vi "teste 9142.vi"() -> ()   [LabVIEW 2018]
uses:
  <vilib>/Instr/_visa.llb/VISA Configure Serial Port (Serial Instr).vi
panel:
  in  "OK Button":bool
  out "read buffer":string
  in  "stop":bool
  in  "Boolean":bool
  in  "read buffer 2":string
  out "error out 2":errorcluster
  in  "VISA resource name":refnum<visa-resource-name>
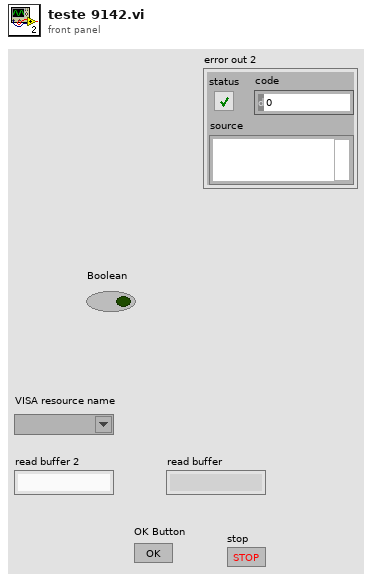
[diagram p1: front panel]
types:
  T1 = enum16{"inserir temp", "carregar temp", "aquisitar temp", "desligar"}
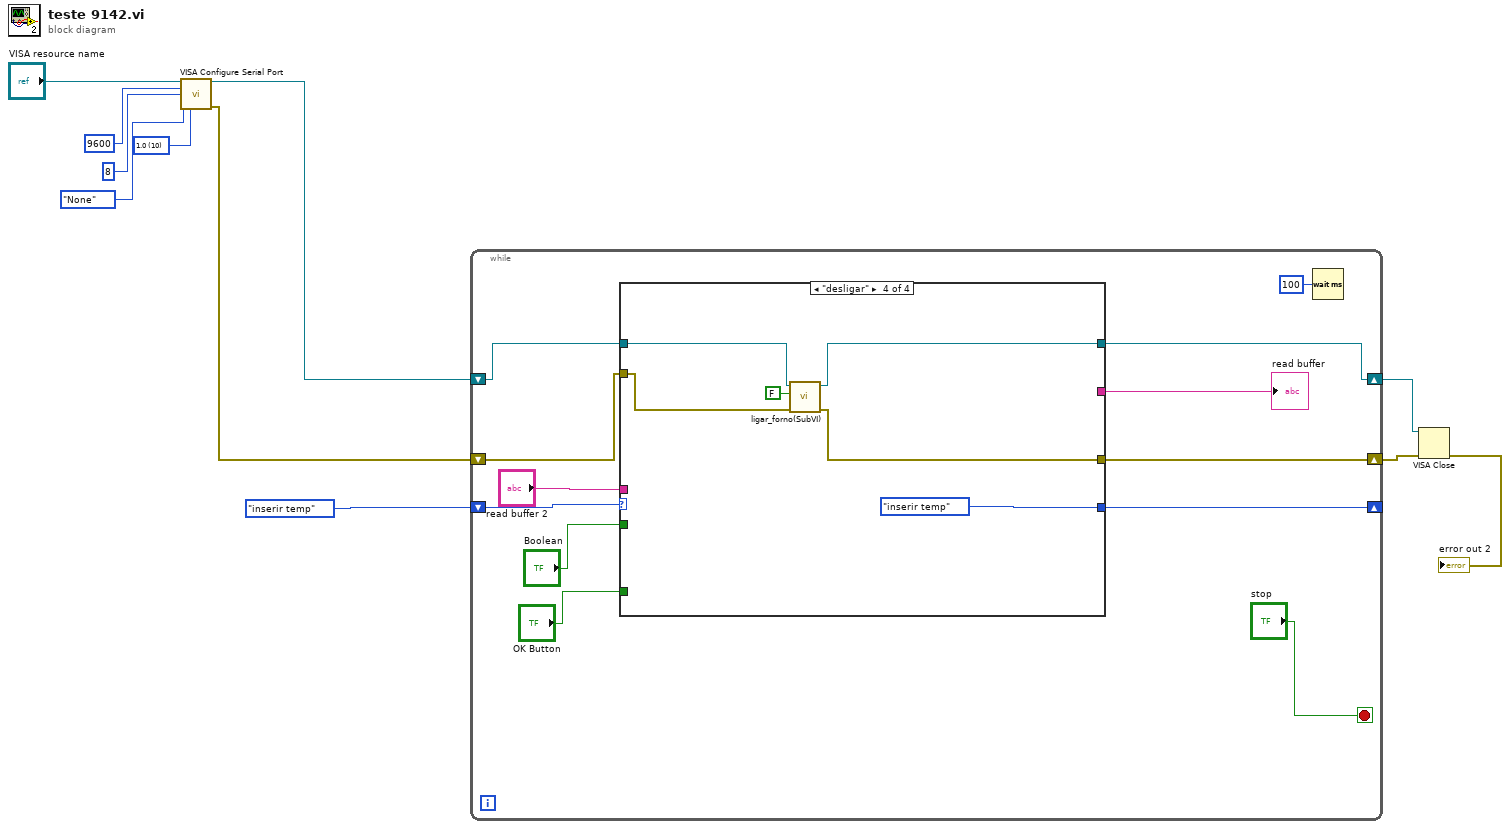
[diagram p0: block diagram]
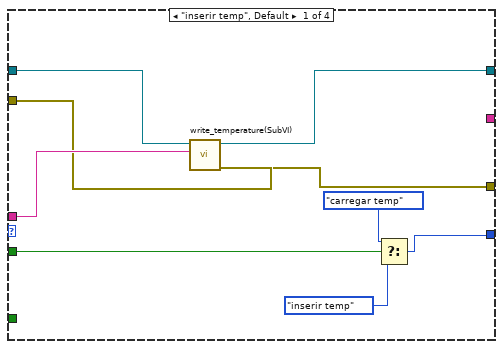
[diagram p2: hidden frame]
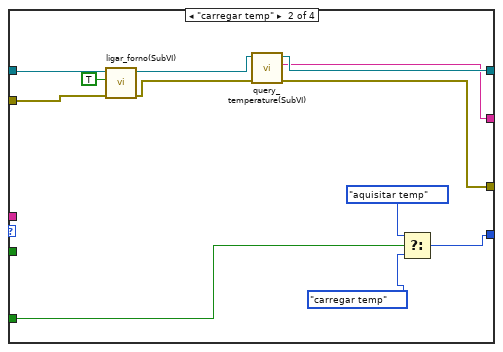
[diagram p3: hidden frame]
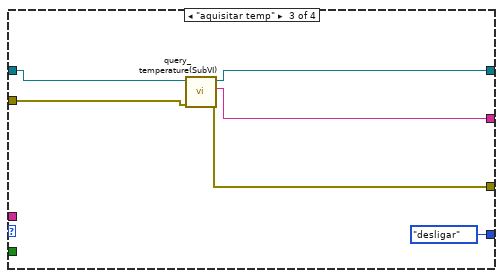
[diagram p4: hidden frame]
diagram:
  w7 = u16 10 items=["1.0"=10, "1.5"=15, "2.0"=20] ("stop bits (10: 1 bit)")
  n1 = call-poly "VISA Configure Serial Port"("VISA resource name"="VISA resource name", "baud rate (9600)"=u32 9600, "data bits (8)"=u16 8, "parity (0:none)"=enum16{"None", "Odd", "Even", "Mark", "Space"}."None", "stop bits (10: 1 bit)"=w7) -> ("VISA resource name out"=w2:refnum<visa-resource-name>, "error out"=w5:errorcluster)  [unwired: 9 in]
  n2 = while {
    shift-right: [w19] -> _
    shift-left: T1."inserir temp" -> [w23]
    shift-right: [w17] -> w4
    shift-left: w5 -> [w18]
    shift-right: [w13] -> w1
    shift-left: w2 -> [w12]
    stop <- "stop" stop-if-true
    n3 = case shown="\"desligar\"" w23 {
      tunnel: "read buffer 2" -> [w32 _ _ _]
      tunnel: "Boolean" -> [w31 _ _ _]
      tunnel: [w30 w42 T1."desligar" T1."inserir temp"] -> w19
      tunnel: w18 -> [w27 w41 w49 w54]
      tunnel: [w26 w36 w48 w55] -> w17
      tunnel: [_ w34 w50 _] -> w16
      tunnel: "OK Button" -> [_ w40 _ _]
      tunnel: [w24 w35 w45 w52] -> w13
      tunnel: w12 -> [w25 w39 w46 w53]
      frame "inserir temp", Default {
        n4 = call "write_temperature(SubVI).vi"("error in (no error)"=w27, "read buffer"=w32, "VISA Refnum in"=w25) -> ("error out"=w26:errorcluster, "VISA resource name out"=w24:refnum<visa-resource-name>)  [unwired: 7 in]
        n5 = Select(t=T1."carregar temp", s=w31, f=T1."inserir temp") -> (s? t:f=w30:T1)
      }
      frame "carregar temp" {
        n6 = call "ligar_forno(SubVI).vi"("error in (no error)"=w41, "s"=TRUE, "VISA Refnum in"=w39) -> ("error out"=w37:errorcluster, "VISA resource name out"=w38:refnum<visa-resource-name>)  [unwired: 7 in]
        n7 = call "query_temperature(SubVI).vi"("error in (no error)"=w37, "VISA Refnum in"=w38) -> ("error out"=w36:errorcluster, "read buffer"=w34:string, "VISA resource name out"=w35:refnum<visa-resource-name>)  [unwired: 7 in]
        n8 = Select(t=T1."aquisitar temp", s=w40, f=T1."carregar temp") -> (s? t:f=w42:T1)
      }
      frame "aquisitar temp" {
        n9 = call "query_temperature(SubVI).vi"("error in (no error)"=w49, "VISA Refnum in"=w46) -> ("error out"=w48:errorcluster, "read buffer"=w50:string, "VISA resource name out"=w45:refnum<visa-resource-name>)  [unwired: 7 in]
      }
      frame "desligar" {
        n10 = call "ligar_forno(SubVI).vi"("error in (no error)"=w54, "s"=FALSE, "VISA Refnum in"=w53) -> ("error out"=w55:errorcluster, "VISA resource name out"=w52:refnum<visa-resource-name>)  [unwired: 7 in]
      }
    }
    "read buffer" <- w16
    n11 = Wait (ms)(milliseconds to wait=u32 100) -> ()  [unwired: 1 out]
  }
  n12 = VISA Close(VISA resource name=w1, error in (no error)=w4) -> (error out=→"error out 2":errorcluster)
